vi "Beta 3.0.1.vi"() -> ()   [LabVIEW 2011]
uses:
  <vilib>/vision/NI_Vision_Development_Module.lvlib
panel:
  in  "Structuring Element":dbl[][](array[numeric])=[[0.0, 1.0, 0.0], [1.0, 1.0, 1.0], [0.0, 1.0, 0.0]]
  in  "Morphology":u16(ring) items=["(none)", "AutoM", "Close", "Dilate", "Erode", "Gradient", "Gradient out", "Gradient in", "Open", "Thick", "Thin"]
  in  "Generate":bool
  in  "Look for":enum16{"Bright Objects", "Dark Objects"}(ring)
  in  "Method":T1(ring)=enum."Inter-class Variance"
  out "Binary":T2(plugin-control)
  out "Threshold Range":cluster{"Lower value":sgl, "Upper value":sgl}={"Lower value"=128.0, "Upper value"=255.0} {"Upper value" format="%.2f"; "Lower value" format="%.2f"}
  in  "Stop":bool
  in  "Browse":bool
  out "XY Graph":cluster{dbl[], dbl[]}(graph)
  out "Original Image":T2(plugin-control)
  out "Path to Image":path
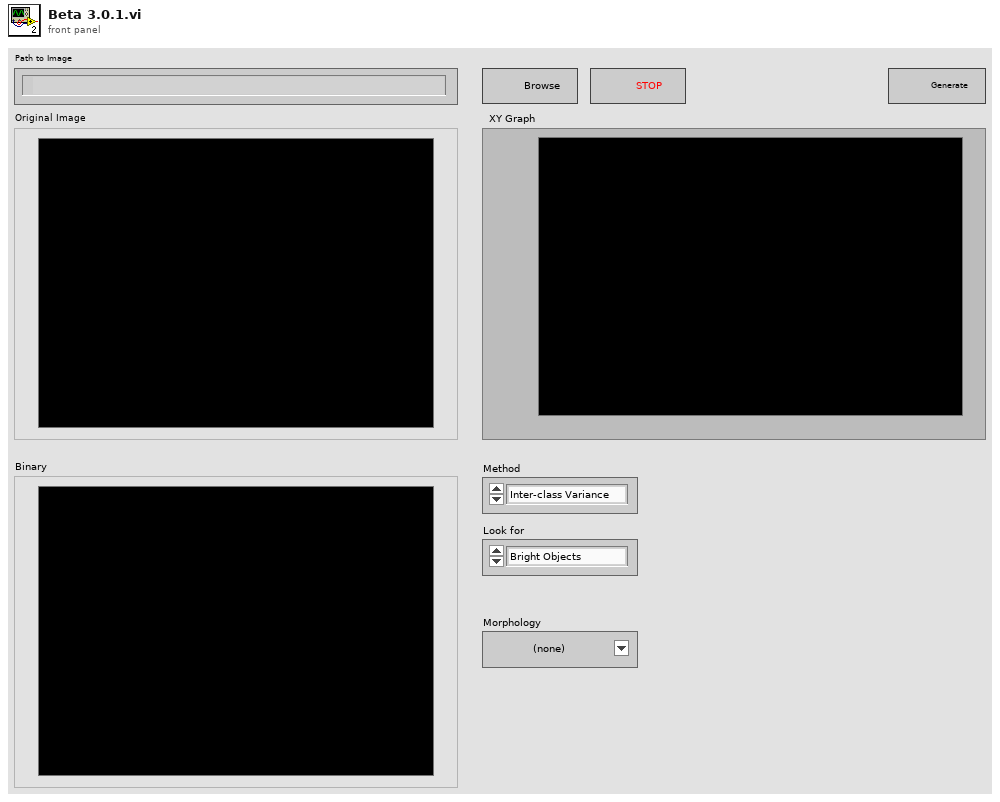
[diagram p1: front panel]
types:
  T1 = enum16{"Clustering", "Entropy", "Metric", "Moments", "Inter-class Variance"}
  T2 = typedef "IMAQ Image.ctl" = refnum<image>
  T3 = typedef "Image Type" = u32
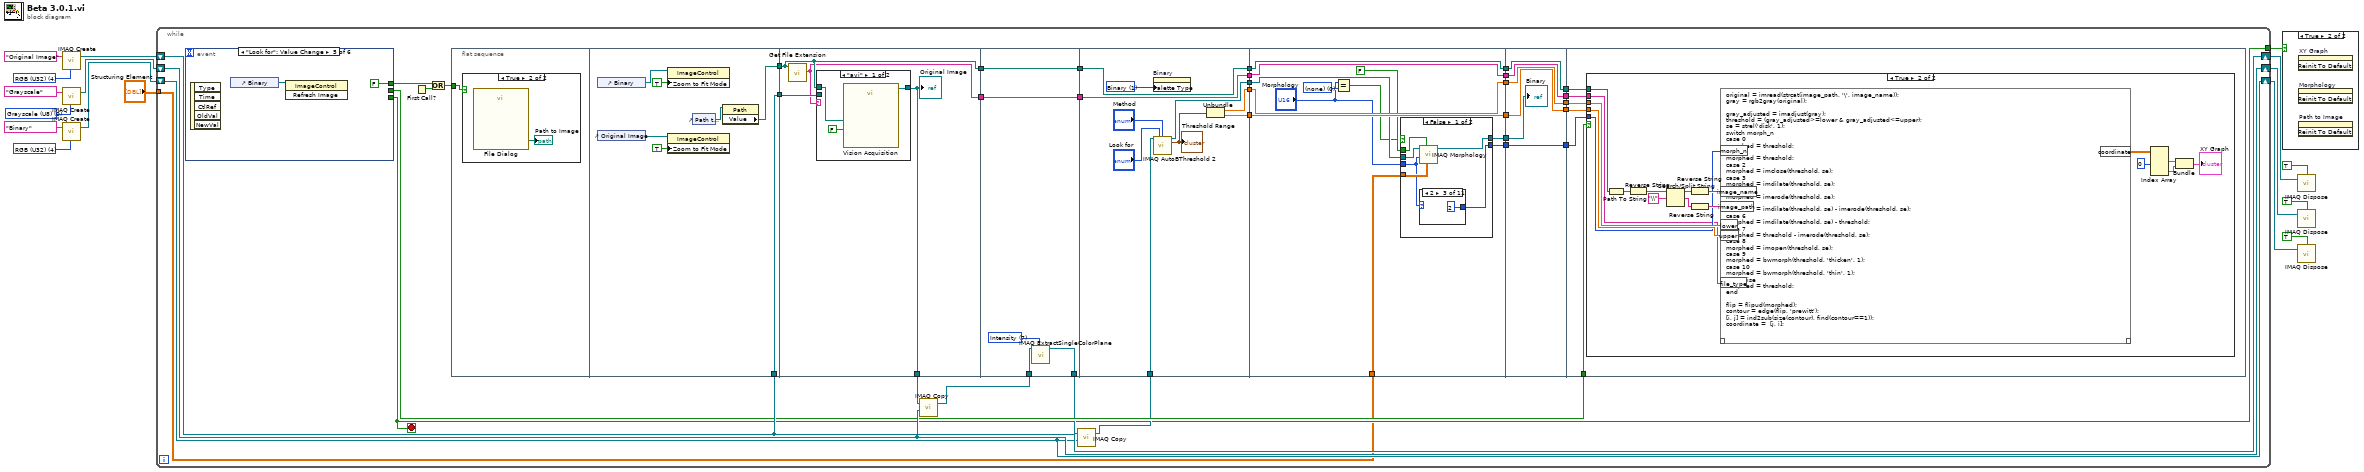
[diagram p0: block diagram]
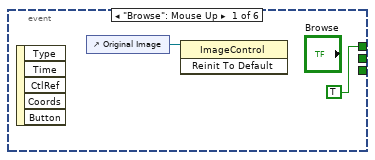
[diagram p3: hidden frame]
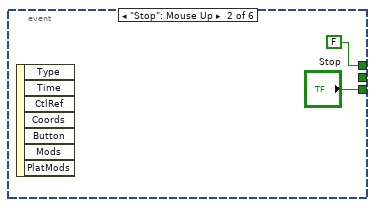
[diagram p4: hidden frame]
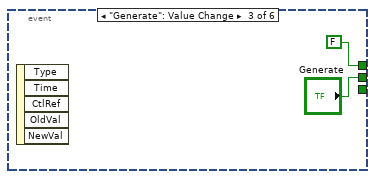
[diagram p5: hidden frame]
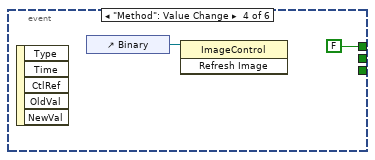
[diagram p6: hidden frame]
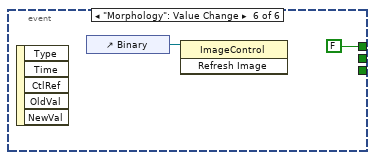
[diagram p7: hidden frame]
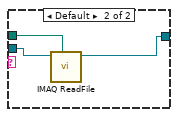
[diagram p9: hidden frame]
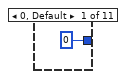
[diagram p10: hidden frame]
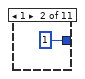
[diagram p11: hidden frame]
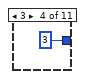
[diagram p12: hidden frame]
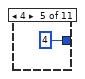
[diagram p13: hidden frame]
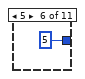
[diagram p14: hidden frame]
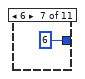
[diagram p15: hidden frame]
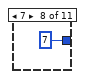
[diagram p16: hidden frame]
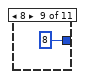
[diagram p17: hidden frame]
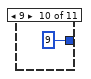
[diagram p18: hidden frame]
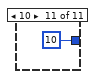
[diagram p19: hidden frame]
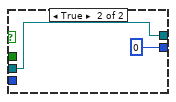
[diagram p20: hidden frame]
diagram:
  w5 = T3 4 items=["Grayscale (U8)", "Grayscale (I16)", "Grayscale (SGL)", "Complex (CSG)", "RGB (U32)", "HSL (U32)", "RGB (U64)", "Grayscale (U16)"] ("Image Type")
  w11 = T3 0 items=["Grayscale (U8)", "Grayscale (I16)", "Grayscale (SGL)", "Complex (CSG)", "RGB (U32)", "HSL (U32)", "RGB (U64)", "Grayscale (U16)"] ("Image Type")
  w16 = T3 4 items=["Grayscale (U8)", "Grayscale (I16)", "Grayscale (SGL)", "Complex (CSG)", "RGB (U32)", "HSL (U32)", "RGB (U64)", "Grayscale (U16)"] ("Image Type")
  n1 = call "IMAQ Create"("Image Name"="Original Image", "Image Type"=w16) -> ("New Image"=w15:T2)  [unwired: 3 in, 1 out]
  n2 = call "IMAQ Create"("Image Name"="Grayscale", "Image Type"=w11) -> ("New Image"=w10:T2)  [unwired: 3 in, 1 out]
  n3 = call "IMAQ Create"("Image Name"="Binary", "Image Type"=w5) -> ("New Image"=w2:T2)  [unwired: 3 in, 1 out]
  n4 = while {
    shift-right: [w47] -> w14
    shift-left: w15 -> [w47]
    tunnel: [w27] -> w13
    shift-right: [w42] -> w8
    shift-left: w10 -> [w42]
    shift-right: [w36] -> w3
    shift-left: w2 -> [w36]
    tunnel: "Structuring Element" -> [w26]
    stop <- w27 stop-if-true
    n5 = event shown="[4] \"Look for\": Value Change" {
      selector: _ -> [_ _ _ _ _ _]
      dyn-events: _ -> [_ _ _ _ _ _]
      timeout: _ -> [_ _ _ _ _ _]
      tunnel: [TRUE FALSE FALSE FALSE FALSE FALSE] -> w51
      tunnel: [_ "Stop" _ _ _ _] -> w27
      tunnel: [_ _ "Generate" _ _ _] -> w41
      event "Browse": Mouse Up {
        n6 = event-data() -> ()  [unwired: 1 in, 5 out]
        n7 = control-ref of="Original Image"() -> (w54:refnum<vi>)
        n8 = invoke class="ImageControl" method="Reinit To Default"(reference=w54) -> ()  [unwired: 2 in, 3 out]
      }
      event "Stop": Mouse Up {
        n9 = event-data() -> ()  [unwired: 1 in, 7 out]
      }
      event "Generate": Value Change {
        n10 = event-data() -> ()  [unwired: 1 in, 5 out]
      }
      event "Method": Value Change {
        n11 = event-data() -> ()  [unwired: 1 in, 5 out]
        n12 = control-ref of="Binary"() -> (w59:refnum<vi>)
        n13 = invoke class="ImageControl" method="Refresh Image"(reference=w59) -> ()  [unwired: 2 in, 3 out]
      }
      event "Look for": Value Change {
        n14 = event-data() -> ()  [unwired: 1 in, 5 out]
        n15 = control-ref of="Binary"() -> (w61:refnum<vi>)
        n16 = invoke class="ImageControl" method="Refresh Image"(reference=w61) -> ()  [unwired: 2 in, 3 out]
      }
      event "Morphology": Value Change {
        n17 = event-data() -> ()  [unwired: 1 in, 5 out]
        n18 = control-ref of="Binary"() -> (w63:refnum<vi>)
        n19 = invoke class="ImageControl" method="Refresh Image"(reference=w63) -> ()  [unwired: 2 in, 3 out]
      }
    }
    n20 = First Call?() -> (First Call?: T/F=w50:bool)
    n21 = Or(x=w51, y=w50) -> (x .or. y?=w49:bool)
    n22 = flat-sequence {
      tunnel: w49 -> [w65]
      tunnel: [w69] -> w52
      tunnel: [w70] -> w48
      tunnel: w47 -> [w69]
      tunnel: w52 -> [w77]
      tunnel: w48 -> [w75]
      tunnel: [w75] -> w46
      tunnel: [w76] -> w23
      tunnel: [w74] -> w18
      tunnel: w46 -> [w88]
      tunnel: [w88] -> w45
      tunnel: w43 -> [w86]
      tunnel: [w85] -> w37
      tunnel: [w84] -> w19
      tunnel: w18 -> [w84]
      tunnel: w45 -> [w98]
      tunnel: [w98] -> w35
      tunnel: [w97] -> w33
      tunnel: [w92] -> w32
      tunnel: [w91] -> w30
      tunnel: w38 -> [w90]
      tunnel: [w89] -> w20
      tunnel: w19 -> [w89]
      tunnel: w35 -> [w110]
      tunnel: [w110] -> w34
      tunnel: w33 -> [w107]
      tunnel: w32 -> [w109]
      tunnel: [w109] -> w31
      tunnel: w30 -> [w108]
      tunnel: [w108] -> w29
      tunnel: [w106] -> w28
      tunnel: w26 -> [w101]
      tunnel: [w100] -> w25
      tunnel: [w99] -> w21
      tunnel: w20 -> [w99]
      tunnel: w34 -> [w135]
      tunnel: [w135] -> w44
      tunnel: [w134] -> w40
      tunnel: w31 -> [w134]
      tunnel: [w133] -> w39
      tunnel: w29 -> [w133]
      tunnel: w28 -> [w132]
      tunnel: w25 -> [w131]
      tunnel: [w131] -> w24
      tunnel: [w130] -> w22
      tunnel: w21 -> [w130]
      tunnel: w44 -> [w141]
      tunnel: w41 -> [w140]
      tunnel: w40 -> [w139]
      tunnel: w39 -> [w138]
      tunnel: w24 -> [w137]
      tunnel: w22 -> [w136]
      frame #0 {
        n23 = case shown="True" w65 {
          frame False {
          }
          frame True {
            n24 = call "File Dialog"() -> ("selected path"=→"Path to Image":path)  [unwired: 12 in, 3 out]
          }
        }
      }
      frame #1 {
        n25 = control-ref of="Binary"() -> (w68:refnum<vi>)
        n26 = control-ref of="Original Image"() -> (w73:refnum<vi>)
        n27 = property class="ImageControl"(reference=w68, "Zoom to Fit Mode"=TRUE) -> ()  [unwired: 1 in, 2 out]
        n28 = property class="ImageControl"(reference=w73, "Zoom to Fit Mode"=TRUE) -> ()  [unwired: 1 in, 2 out]
        n29 = control-ref of="Path to Image"() -> (w71:refnum<vi>)
        n30 = property class="Path"(reference=w71) -> ("Value"=w70:path)  [unwired: 1 in, 2 out]
      }
      frame #2 {
        n31 = call <vilib>:"Get File Extension.vi"("file"=w75) -> ("lowercase file extension"=w74:string)  [unwired: 7 in, 3 out]
        n32 = case shown="\"avi\"" w74 {
          tunnel: w77 -> [_ w83]
          tunnel: w75 -> [w80 w82]
          tunnel: [w79 w81] -> w76
          frame "avi" {
            n33 = call "Vision Acquisition"("AVI Path"=w80, "Stop (F)"=FALSE) -> ("Image Out"=w79:T2)  [unwired: 1 in, 24 out]
          }
          frame Default {
            n34 = call "IMAQ ReadFile"("File Path"=w82, "Image"=w83) -> ("Image Out"=w81:T2)  [unwired: 5 in, 4 out]
          }
        }
        "Original Image" <- w76
      }
      frame #3 {
        w87 = 7 items=["Red", "Green", "Blue", "Hue", "Saturation", "Luminance", "Value", "Intensity"] ("Color Plane")
        n35 = call "IMAQ ExtractSingleColorPlane"("Color Plane"=w87, "Image Src"=w86) -> ("Image Dst Out"=w85:T2)  [unwired: 8 in, 1 out]
      }
      frame #4 {
        w96 = u32 1 items=["Grayscale", "Binary", "Gradient", "Rainbow", "Temperature", "User Defined"] ("Palette")
        n36 = property on="Binary" class="ImageControl"("Palette Type"=w96) -> ()  [unwired: 2 in, 2 out]
        n37 = call "IMAQ AutoBThreshold 2"("Image Src"=w90, "Look For (Bright Objects)"="Look for", "Method (clustering)"="Method") -> ("Image Dst Out"=w97:T2, "Threshold Range Out"=w93:cluster{"Lower value":sgl, "Upper value":sgl})  [unwired: 10 in, 1 out]
        "Threshold Range" <- w93
        n38 = Unbundle(w93) -> ("Lower value"=w92:sgl, "Upper value"=w91:sgl)
      }
      frame #5 {
        w104 = u16 0 items=["(none)"]
        n39 = Equal?(x="Morphology", y=w104) -> (x = y?=w103:bool)
        n40 = case shown="False" w103 {
          tunnel: w107 -> [w114 w129]
          tunnel: [w115 w129] -> w106
          tunnel: FALSE -> [w116 _]
          tunnel: "Morphology" -> [w112 _]
          tunnel: w101 -> [w113 _]
          tunnel: [w111 0] -> w100
          frame False {
            n41 = call "IMAQ Morphology"("Structuring Element"=w113, "Square/Hexa (Square)"=w116, "Operation"=w112, "Image Src"=w114) -> ("Image Dst Out"=w115:T2)  [unwired: 6 in, 1 out]
            n42 = case shown="2" w112 {
              tunnel: [0 1 2 3 4 5 6 7 8 9 10] -> w111
              frame 0, Default {
              }
              frame 1 {
              }
              frame 2 {
              }
              frame 3 {
              }
              frame 4 {
              }
              frame 5 {
              }
              frame 6 {
              }
              frame 7 {
              }
              frame 8 {
              }
              frame 9 {
              }
              frame 10 {
              }
            }
          }
          frame True {
          }
        }
      }
      frame #6 {
        "Binary" <- w132
      }
      frame #7 {
        n43 = case shown="True" w140 {
          tunnel: w141 -> [_ w158]
          tunnel: w139 -> [_ w145]
          tunnel: w138 -> [_ w144]
          tunnel: w137 -> [_ w143]
          tunnel: w136 -> [_ w142]
          frame False {
          }
          frame True {
            n44 = Path To String(path=w158) -> (string=w157:string)
            n45 = Reverse String(1:w157) -> (0:w156:string)
            n46 = Search/Split String(string=w156, search string/char (-)="\\") -> (substring before match=w154:string, match + rest of string=w153:string)  [unwired: 1 in, 1 out]
            n47 = Reverse String(1:w154) -> (0:w152:string)
            n48 = Reverse String(1:w153) -> (0:w151:string)
            n49 = script code="original = imread(strcat(image_path, '\\', image_name));\ngray = rgb2gray(original);\n\ngray_adjusted = imadjust(gray);\nthreshold = (gray_adjusted>=lower & gray_adjusted<=upper);\nse = strel('disk', 1);\nswitch morph_n\ncase 0\nmorphed = threshold;\ncase 1\nmorphed = threshold;\ncase 2\nmorphed = imclose(threshold, se);\ncase 3\nmorphed = imdilate(threshold, se);\ncase 4\nmorphed = imerode(threshold, se);\ncase 5\nmorphed = imdilate(threshold, se) - imerode(threshold, se);\ncase 6\nmorphed = imdilate(threshold, se) - threshold;\ncase 7\nmorphed = threshold - imerode(threshold, se);\ncase 8\nmorphed = imopen(threshold, se);\ncase 9\nmorphed = bwmorph(threshold, 'thicken', 1);\ncase 10\nmorphed = bwmorph(threshold, 'thin', 1);\notherwise\nmorphed = threshold;\nend\n\nflip = flipud(morphed);\ncontour = edge(flip, 'prewitt');\n[i, j] = ind2sub(size(contour), find(contour==1));\ncoordinate =  [j, i];"("image_name"=w152, "image_path"=w151, "lower"=w145, "upper"=w144, "morph_n"=w143, "file_type"=w142) -> ("coordinate"=w150:dbl[][])  [unwired: 1 in, 1 out]
            n50 = Index Array(array=w150, index (col) #1=0 ("disabled index (col)")) -> (element #1=w149:dbl[], element #2=w148:dbl[])  [unwired: 3 in]
            n51 = Bundle(w149, w148) -> (→"XY Graph":cluster{dbl[], dbl[]})  [unwired: 1 in]
          }
        }
      }
    }
    n52 = call "IMAQ Copy"("Image Dst"=w42, "Image Src"=w23) -> ("Image Dst Out"=w43:T2)  [unwired: 4 in, 1 out]
    n53 = call "IMAQ Copy"("Image Dst"=w36, "Image Src"=w37) -> ("Image Dst Out"=w38:T2)  [unwired: 4 in, 1 out]
  }
  n54 = case shown="True" w13 {
    frame False {
    }
    frame True {
      n55 = invoke on="XY Graph" class="XYGraph (strict)" method="Reinit To Default"() -> ()  [unwired: 3 in, 3 out]
      n56 = invoke on="Morphology" class="Ring (strict)" method="Reinit To Default"() -> ()  [unwired: 3 in, 3 out]
      n57 = invoke on="Path to Image" class="Path" method="Reinit To Default"() -> ()  [unwired: 3 in, 3 out]
    }
  }
  n58 = call "IMAQ Dispose"("All Images? (No)"=TRUE, "Image"=w14) -> ()  [unwired: 4 in, 1 out]
  n59 = call "IMAQ Dispose"("All Images? (No)"=TRUE, "Image"=w8) -> ()  [unwired: 4 in, 1 out]
  n60 = call "IMAQ Dispose"("All Images? (No)"=TRUE, "Image"=w3) -> ()  [unwired: 4 in, 1 out]
